vi "Calc Drive.vi"(3 "Target Speed":dbl(slide) scale=-0.75..0.75, 4 "Rate Right":dbl, 5 "Rate Left":dbl) -> (0 "Y Out":dbl, 1 "X Out":dbl)   [LabVIEW 2015]
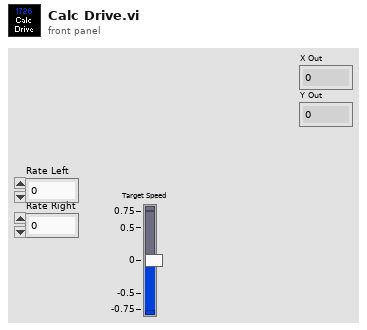
[diagram p1: front panel]
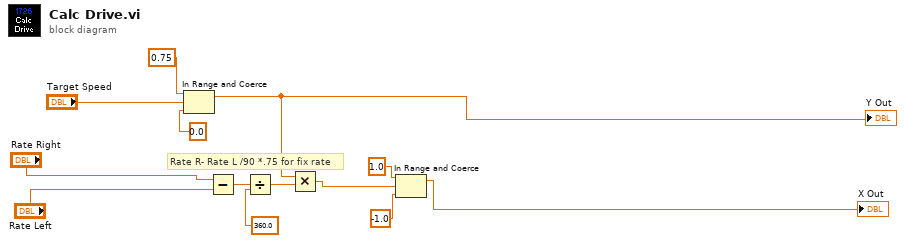
[diagram p0: block diagram]
diagram:
  # "Rate R- Rate L /90 *.75 for fix rate"
  n1 = In Range and Coerce(upper limit=0.75, x="Target Speed", lower limit=0.0) -> (coerced(x)=w1:dbl)  [unwired: 1 out]
  "Y Out" <- w1
  n2 = Subtract(x="Rate Right", y="Rate Left") -> (x-y=w8:dbl)
  n3 = Divide(x=w8, y=360.0) -> (x/y=w6:dbl)
  n4 = Multiply(x=w1, y=w6) -> (x*y=w4:dbl)
  n5 = In Range and Coerce(upper limit=1.0, x=w4, lower limit=-1.0) -> (coerced(x)=→"X Out":dbl)  [unwired: 1 out]
